vi "Call_Block_plug_ins.vi"(0 "Per Block Plug Ins":string[](array[string])) -> ()   [LabVIEW 2011]
uses:
  Globals/Dynamic_call_global.ph.vi
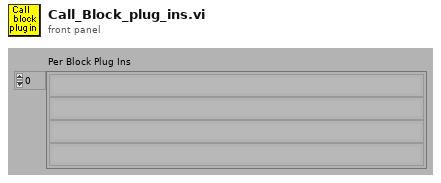
[diagram p1: front panel]
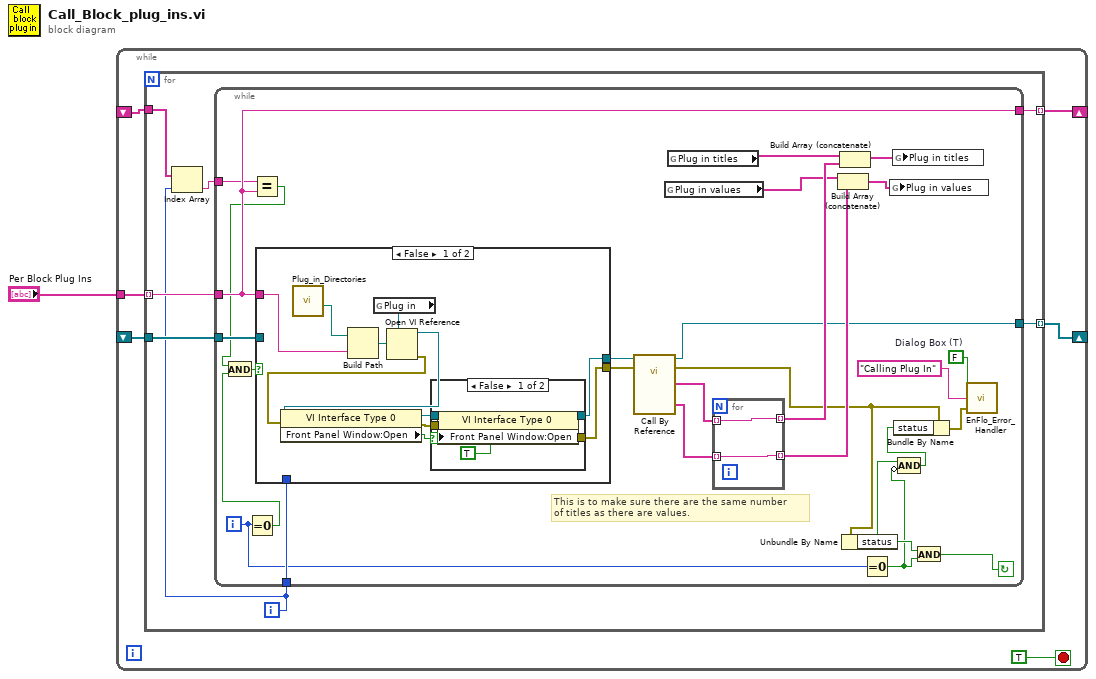
[diagram p0: block diagram]
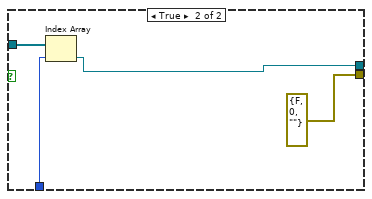
[diagram p3: hidden frame]
diagram:
  n1 = while {
    tunnel: "Per Block Plug Ins" -> [w7]
    shift-right: [w6] -> _
    shift-left: _ -> [w5]
    shift-right: [w3] -> _
    shift-left: _ -> [w2]
    stop <- TRUE stop-if-true
    n2 = for {
      tunnel: w7 -> [w14] mode=indexing
      tunnel: [w13] -> w6 mode=indexing
      tunnel: w5 -> [w12]
      tunnel: [w11] -> w3 mode=indexing
      tunnel: w2 -> [w9]
      i -> [w10]
      n3 = Index Array(array=w9, index=w10) -> (element=w8:string)
      n4 = while {
        tunnel: w14 -> [w23]
        tunnel: [w35] -> w13
        tunnel: w10 -> [w34]
        tunnel: w12 -> [w33]
        tunnel: [w23] -> w11
        tunnel: w8 -> [w22]
        i -> [w24]
        stop <- w30 continue-if-true
        w32 = FALSE  # Dialog Box (T)
        # "This is to make sure there are the same number\nof titles as there are values."
        n5 = Equal To 0?(x=w24) -> (x = 0?=w20:bool)
        n6 = Equal?(x=w22, y=w23) -> (x = y?=w19:bool)
        n7 = And(x=w19, y=w20) -> (x .and. y?=w21:bool)
        n8 = case shown="False" w21 {
          tunnel: [w45 errorcluster {"status"=FALSE, "code"=0, "source"=""} ("error out")] -> w37
          tunnel: [w43 w61] -> w36
          tunnel: w23 -> [w42 _]
          tunnel: w34 -> [_ w63]
          tunnel: w33 -> [_ w62]
          frame False {
            n9 = call "Plug_in_Directories.vi"() -> ("Per Block"=w52:path)  [unwired: 3 out]
            n10 = Build Path(base path=w52, name or relative path=w42) -> (appended path=w44:path)
            n11 = global read "Dynamic_call_global.ph.vi" "Plug in"() -> (w51:refnum<vi>)
            n12 = Open VI Reference(type specifier VI Refnum (for type only)=w51, vi path=w44) -> (vi reference=w50:refnum<vi>, error out=w49:errorcluster)  [unwired: 2 in, 2 out]
            n13 = property class="VI Interface Type 0"(reference=w50, error in=w49) -> (reference out=w47:refnum<vi>, error out=w46:errorcluster, "Front Panel Window:Open"=w48:bool)
            n14 = case shown="False" w48 {
              tunnel: w47 -> [w57 w59]
              tunnel: w46 -> [w56 w58]
              tunnel: [w55 w59] -> w43
              tunnel: [w53 w58] -> w45
              frame False {
                n15 = property class="VI Interface Type 0"(reference=w57, error in=w56, "Front Panel Window:Open"=TRUE) -> (reference out=w55:refnum<vi>, error out=w53:errorcluster)
              }
              frame True {
              }
            }
          }
          frame True {
            n16 = Index Array(array=w62, index=w63) -> (element=w61:refnum<vi>)
          }
        }
        n17 = call-by-ref "?"(reference=w36, error in=w37) -> (reference out=w35:refnum<vi>, error out=w29:errorcluster, "Plug in titles"=w40:string[], "Plug in values"=w38:string[])  [unwired: 6 in]
        n18 = global read "Dynamic_call_global.ph.vi" "Plug in values"() -> (w18:string[])
        n19 = global read "Dynamic_call_global.ph.vi" "Plug in titles"() -> (w17:string[])
        n20 = for {
          tunnel: [w65] -> w41 mode=indexing
          tunnel: w40 -> [w65] mode=indexing
          tunnel: [w64] -> w39 mode=indexing
          tunnel: w38 -> [w64] mode=indexing
        }
        n21 = Build Array (concatenate)(w18, w39) -> (w16:string[])
        n22 = Build Array (concatenate)(w17, w41) -> (w15:string[])
        n23 = Unbundle By Name(w29) -> ("status"=w27:bool)
        n24 = Equal To 0?(x=w24) -> (x = 0?=w26:bool)
        n25 = global write "Dynamic_call_global.ph.vi" "Plug in values"(w16) -> ()
        n26 = global write "Dynamic_call_global.ph.vi" "Plug in titles"(w15) -> ()
        n27 = Compound Arithmetic op=AND(w27, invert w26) -> (w25:bool)
        n28 = Bundle By Name(cluster=w29, "status"=w25) -> (w28:errorcluster)
        n29 = And(x=w27, y=w26) -> (x .and. y?=w30:bool)
        n30 = call "EnFlo_Error_Handler.vi"("error in (no error)"=w28, "Error Type"="Calling Plug In", "Dialog Box (T)"=w32) -> ()  [unwired: 3 out]
      }
    }
  }
